vi "Set Configurable Device Parameter - PulseWidthStep.vi"(2 "IPG_Magnet_Options New Value":string="1234", 3 "Get Configurable Device Parameters read from Zarlink":string) -> (0 "IPG_Magnet_Options Old Value":string="100", 1 "Set Configurable Device Parameters to send to Zarlink":string)   [LabVIEW 2010]
doc: "This VI expects a (\\r\\n) line-terminated multipline String composed of Key = Value pairs, such as:\n\naKey1=value1(\\r\\n)\naKey2=value2(\\r\\n)\n.......\n\nNew Value is the replacement value for the Key.\nOld Value is the value that was initial found before being replaced.\n\nRM 08/12/2013"
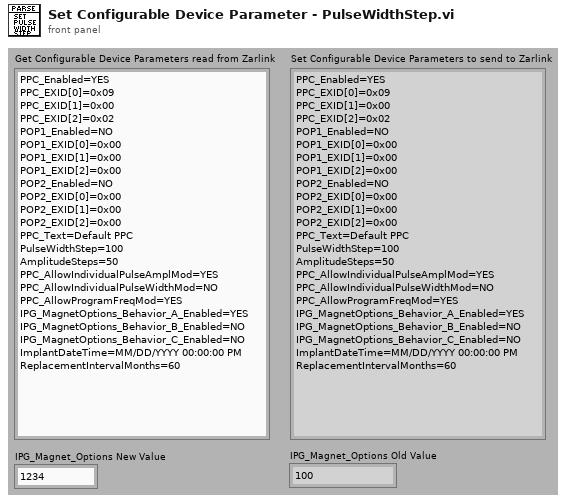
[diagram p1: front panel]
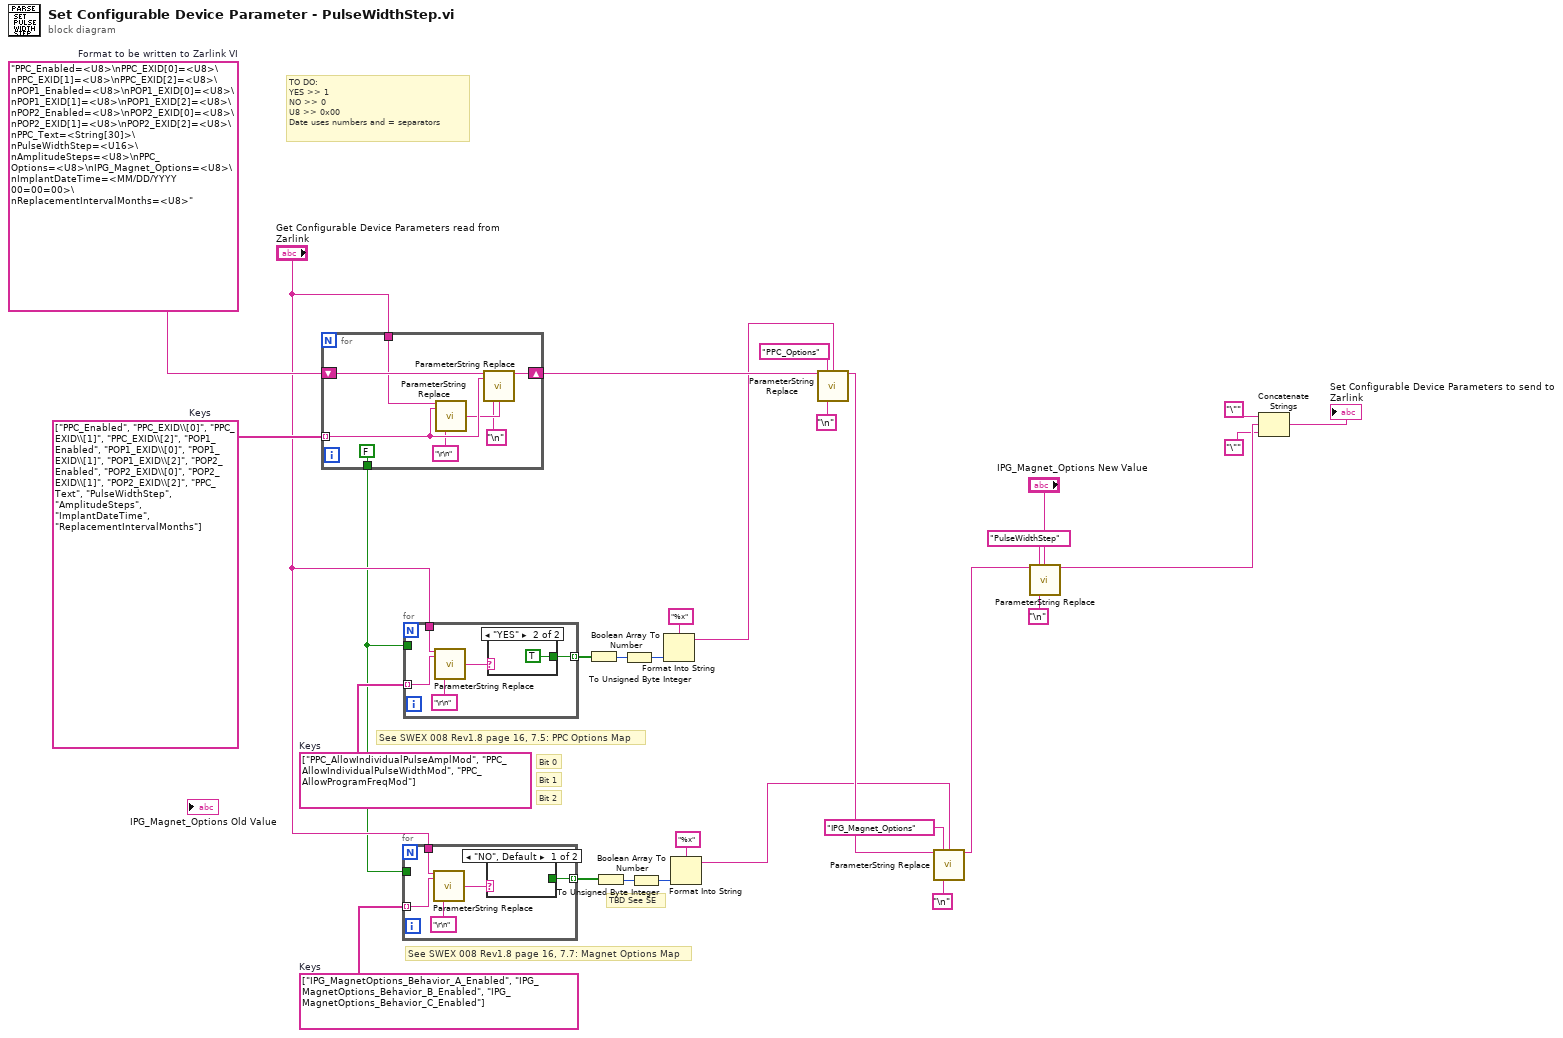
[diagram p0: block diagram]
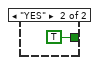
[diagram p2: hidden frame]
diagram:
  w26 = string[] ["IPG_MagnetOptions_Behavior_A_Enabled", "IPG_MagnetOptions_Behavior_B_Enabled", "IPG_MagnetOptions_Behavior_C_Enabled"]  # Keys
  w28 = string[] ["PPC_AllowIndividualPulseAmplMod", "PPC_AllowIndividualPulseWidthMod", "PPC_AllowProgramFreqMod"]  # Keys
  w30 = string[] ["PPC_Enabled", "PPC_EXID\\[0]", "PPC_EXID\\[1]", "PPC_EXID\\[2]", "POP1_Enabled", "POP1_EXID\\[0]", "POP1_EXID\\[1]", "POP1_EXID\\[2]", "POP2_Enabled", "POP2_EXID\\[0]", "POP2_EXID\\[1]", "POP2_EXID\\[2]", "PPC_Text", "PulseWidthStep", "AmplitudeSteps", "ImplantDateTime", "ReplacementIntervalMonths"]  # Keys
  w29 = "PPC_Enabled=<U8>\nPPC_EXID[0]=<U8>\nPPC_EXID[1]=<U8>\nPPC_EXID[2]=<U8>\nPOP1_Enabled=<U8>\nPOP1_EXID[0]=<U8>\nPOP1_EXID[1]=<U8>\nPOP1_EXID[2]=<U8>\nPOP2_Enabled=<U8>\nPOP2_EXID[0]=<U8>\nPOP2_EXID[1]=<U8>\nPOP2_EXID[2]=<U8>\nPPC_Text=<String[30]>\nPulseWidthStep=<U16>\nAmplitudeSteps=<U8>\nPPC_Options=<U8>\nIPG_Magnet_Options=<U8>\nImplantDateTime=<MM/DD/YYYY 00=00=00>\nReplacementIntervalMonths=<U8>"  # Format to be written to Zarlink VI
  # "TO DO:\nYES >> 1\nNO >> 0\nU8 >> 0x00\nDate uses numbers and = separators"
  # "See SWEX 008 Rev1.8 page 16, 7.7: Magnet Options Map"
  # "TBD See SE"
  # "See SWEX 008 Rev1.8 page 16, 7.5: PPC Options Map"
  # "Bit 2"
  # "Bit 1"
  # "Bit 0"
  n1 = for {
    shift-right: [w36] -> w22
    shift-left: w29 -> [w38]
    tunnel: w30 -> [w37] mode=indexing
    tunnel: "Get Configurable Device Parameters read from Zarlink" -> [w32]
    tunnel: [FALSE] -> w5
    n2 = call "ParameterString Replace.vi"("String"=w32, "Key"=w37, "TermChars"="\r\n") -> ("Old Value"=w35:string)  [unwired: 10 in, 2 out]
    n3 = call "ParameterString Replace.vi"("String"=w38, "Key"=w37, "New Value"=w35, "TermChars"="\n") -> ("Updated String"=w36:string)  [unwired: 9 in, 2 out]
  }
  n4 = for {
    tunnel: w26 -> [w43] mode=indexing
    tunnel: "Get Configurable Device Parameters read from Zarlink" -> [w41]
    tunnel: [w39] -> w14 mode=indexing
    tunnel: w5 -> [_]
    n5 = call "ParameterString Replace.vi"("String"=w41, "Key"=w43, "TermChars"="\r\n") -> ("Old Value"=w40:string)  [unwired: 10 in, 2 out]
    n6 = case shown="\"NO\", Default" w40 {
      tunnel: [_ TRUE] -> w39
      frame "NO", Default {
      }
      frame "YES" {
      }
    }
  }
  n7 = for {
    tunnel: w28 -> [w49] mode=indexing
    tunnel: "Get Configurable Device Parameters read from Zarlink" -> [w47]
    tunnel: [w45] -> w25 mode=indexing
    tunnel: w5 -> [_]
    n8 = call "ParameterString Replace.vi"("String"=w47, "Key"=w49, "TermChars"="\r\n") -> ("Old Value"=w46:string)  [unwired: 10 in, 2 out]
    n9 = case shown="\"YES\"" w46 {
      tunnel: [_ TRUE] -> w45
      frame "NO", Default {
      }
      frame "YES" {
      }
    }
  }
  n10 = Boolean Array To Number(Boolean array=w25) -> (number=w24:u32)
  n11 = Boolean Array To Number(Boolean array=w14) -> (number=w15:u32)
  n12 = To Unsigned Byte Integer(number=w24) -> (unsigned 8bit integer=w20:u8)
  n13 = To Unsigned Byte Integer(number=w15) -> (unsigned 8bit integer=w16:u8)
  n14 = Format Into String(format string="%x", w20) -> (resulting string=w18:string)  [unwired: 2 in, 1 out]
  n15 = Format Into String(format string="%x", w16) -> (resulting string=w10:string)  [unwired: 2 in, 1 out]
  n16 = call "ParameterString Replace.vi"("String"=w22, "Key"="PPC_Options", "New Value"=w18, "TermChars"="\n") -> ("Updated String"=w11:string)  [unwired: 9 in, 2 out]
  n17 = call "ParameterString Replace.vi"("String"=w11, "Key"="IPG_Magnet_Options", "New Value"=w10, "TermChars"="\n") -> ("Updated String"=w6:string)  [unwired: 9 in, 2 out]
  n18 = call "ParameterString Replace.vi"("String"=w6, "Key"="PulseWidthStep", "New Value"="IPG_Magnet_Options New Value", "TermChars"="\n") -> ("Updated String"=w4:string)  [unwired: 9 in, 2 out]
  n19 = Concatenate Strings("\"", w4, "\"") -> (→"Set Configurable Device Parameters to send to Zarlink":string)
